vi "add transfer to group.vi"(8 "error in (no error)":errorcluster, 9 "transfer id":string, 10 "id":string, 11 "DSFConfiguration in":refnum<class "DSFConfiguration.lvclass">) -> (0 "error out":errorcluster, 3 "DSFConfiguration out":refnum<class "DSFConfiguration.lvclass">)   [LabVIEW 2017, in "DSFConfiguration.lvclass"]
uses:
  DSFConfiguration.lvclass
  DSFConfiguration.lvclass/DSFConfiguration.ctl
  DSFGroup/DSFGroup.lvclass/DSFGroup.ctl
  DSFGroup/Write transfer ids.vi
  DSFGroup/Read transfer ids.vi
  DSFGroup/DSFGroup.lvclass
  C:/github/data-sharing-framework/Source/Configuration API/Classes/IDable/IDable.lvclass
  DSFTransfer/DSFTransfer.lvclass
  ID API/ID API.lvclass
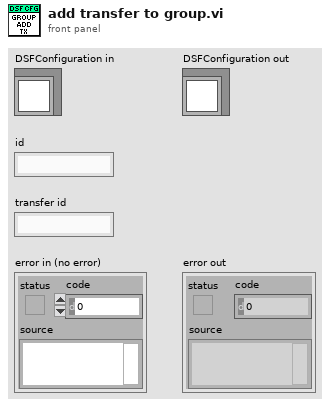
[diagram p1: front panel]
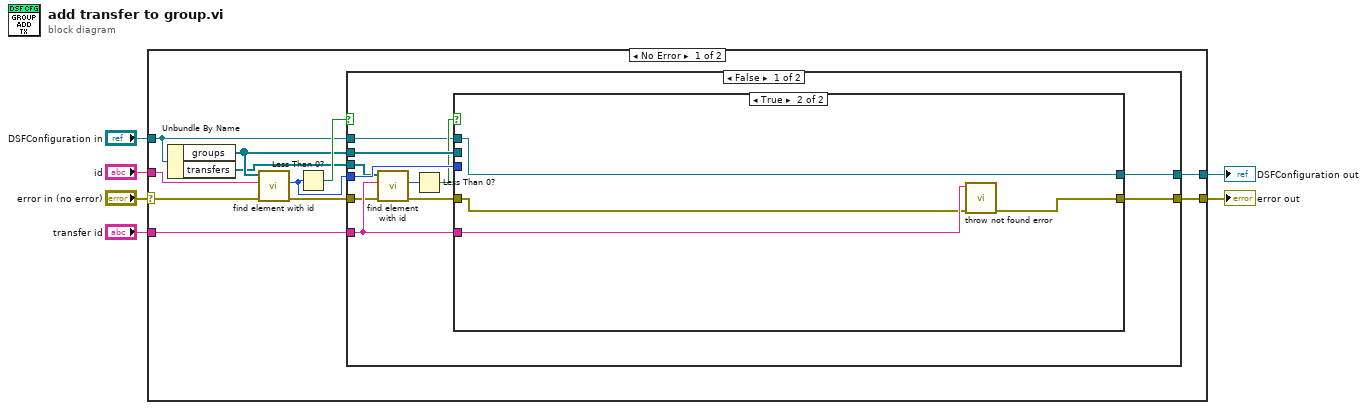
[diagram p0: block diagram]
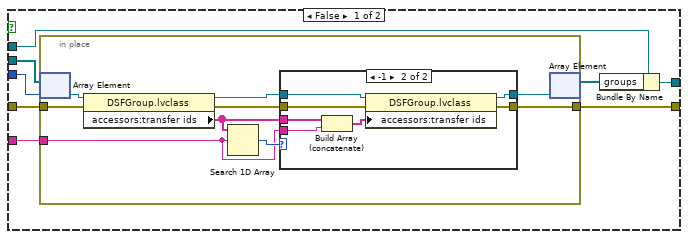
[diagram p2: hidden frame]
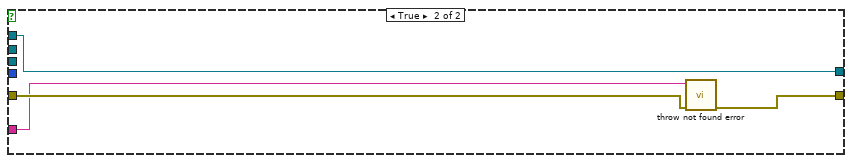
[diagram p4: hidden frame]
diagram:
  n1 = case shown="No Error" "error in (no error)" {
    selector: "error in (no error)" -> [w16 w64]
    tunnel: [w15 w64] -> w5
    tunnel: [w7 w63] -> w3
    tunnel: "DSFConfiguration in" -> [w8 w63]
    tunnel: "id" -> [w17 _]
    tunnel: "transfer id" -> [w14 _]
    frame No Error {
      n2 = Unbundle By Name(w8) -> ("groups"=w11:refnum<class "DSFGroup.lvclass">[], "transfers"=w9:refnum<class "DSFTransfer.lvclass">[])
      n3 = call "find element with id.vi"("error in (no error)"=w16, "id"=w17, "IDable Array in"=w11) -> ("error out"=w12:errorcluster, "index"=w10:i32)  [unwired: 7 in]
      n4 = Less Than 0?(x=w10) -> (x < 0?=w13:bool)
      n5 = case shown="False" w13 {
        tunnel: w12 -> [w19 w60]
        tunnel: [w26 w62] -> w15
        tunnel: w11 -> [w28 _]
        tunnel: w10 -> [w27 _]
        tunnel: w14 -> [w24 w59]
        tunnel: [w25 w61] -> w7
        tunnel: w9 -> [w23 _]
        tunnel: w8 -> [w20 w61]
        frame False {
          n6 = call "find element with id.vi"("error in (no error)"=w19, "id"=w24, "IDable Array in"=w23) -> ("error out"=w18:errorcluster, "index"=w22:i32)  [unwired: 7 in]
          n7 = Less Than 0?(x=w22) -> (x < 0?=w21:bool)
          n8 = case shown="True" w21 {
            tunnel: w28 -> [w35 _]
            tunnel: w27 -> [w34 _]
            tunnel: w18 -> [w33 w55]
            tunnel: [w31 w58] -> w26
            tunnel: [w30 w57] -> w25
            tunnel: w24 -> [w32 w56]
            tunnel: w20 -> [w29 w57]
            frame False {
              n9 = in-place {
                in-place-border: w32 -> [w41]
                in-place-border: w33 -> [w44]
                in-place-border: [w38] -> w31
                n10 = in-place-array #1(w35, w34) -> (w45:refnum<class "DSFGroup.lvclass">)
                n11 = property class="DSFGroup.lvclass"(reference=w45, error in=w44) -> (reference out=w40:refnum<class "DSFGroup.lvclass">, error out=w39:errorcluster, "accessors:transfer ids"=w42:string[])
                n12 = Search 1D Array(1D array=w42, element=w41) -> (index of element=w43:i32)  [unwired: 1 in]
                n13 = case shown="-1" w43 {
                  tunnel: w42 -> [_ w54]
                  tunnel: w41 -> [_ w53]
                  tunnel: w40 -> [w47 w52]
                  tunnel: w39 -> [w46 w51]
                  tunnel: [w46 w50] -> w38
                  tunnel: [w47 w49] -> w37
                  frame Default {
                  }
                  frame -1 {
                    n14 = Build Array (concatenate)(w54, w53) -> (w48:string[])
                    n15 = property class="DSFGroup.lvclass"(reference=w52, error in=w51, "accessors:transfer ids"=w48) -> (reference out=w49:refnum<class "DSFGroup.lvclass">, error out=w50:errorcluster)
                  }
                }
                n16 = in-place-array #1(w37) -> (w36:refnum<class "DSFGroup.lvclass">[])  [unwired: 1 out]
              }
              n17 = Bundle By Name(cluster=w29, "groups"=w36) -> (w30:refnum<class "DSFConfiguration.lvclass">)
            }
            frame True {
              n18 = call "throw not found error.vi"("error in (no error)"=w55, "id"=w56) -> ("error out"=w58:errorcluster)  [unwired: 9 in]
            }
          }
        }
        frame True {
          n19 = call "throw not found error.vi"("error in (no error)"=w60, "id"=w59) -> ("error out"=w62:errorcluster)  [unwired: 9 in]
        }
      }
    }
    frame Error {
    }
  }
  "error out" <- w5
  "DSFConfiguration out" <- w3
